vi "LV connector pane.vi"(8 "error in (no error)":errorcluster, 11 "reference":refnum<vi>) -> (0 "error out":errorcluster, 3 "conpane":string)   [LabVIEW 2012]
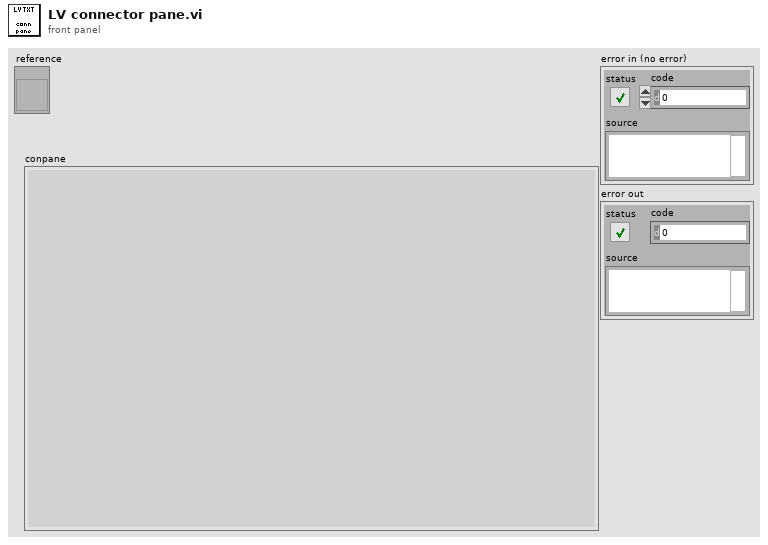
[diagram p1: front panel]
types:
  T1 = enum16{"Invalid Wire Rule", "Required", "Recommended", "Optional", "Dynamic Dispatch"}[]
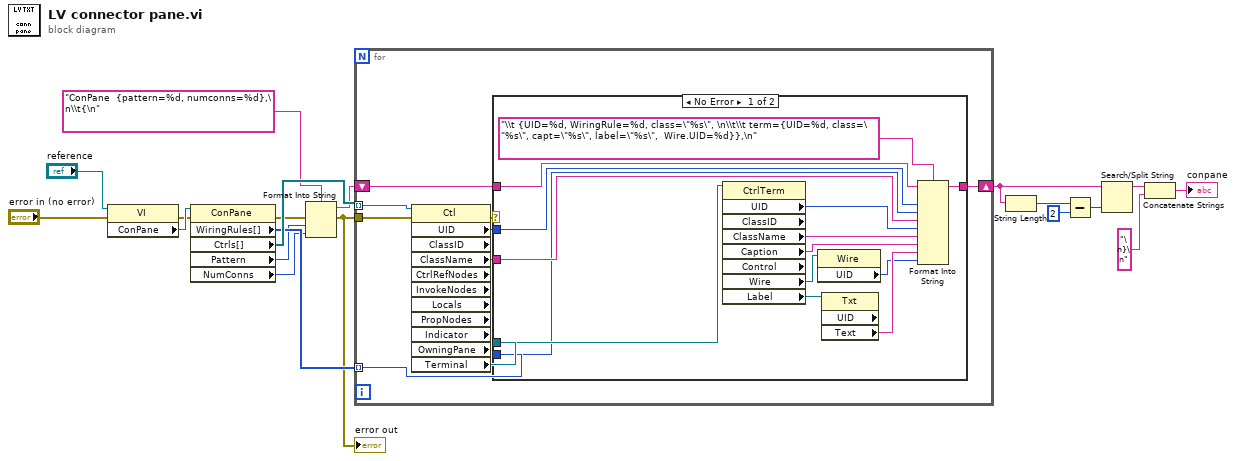
[diagram p0: block diagram]
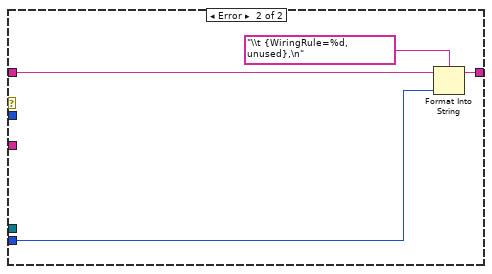
[diagram p2: hidden frame]
diagram:
  n1 = property class="VI"(reference="reference", error in="error in (no error)") -> (error out=w2:errorcluster, "ConPane"=w19:refnum<vi>)  [unwired: 1 out]
  n2 = property class="ConPane"(reference=w19, error in=w2) -> (error out=w5:errorcluster, "WiringRules[]"=w10:T1, "Ctrls[]"=w11:refnum<vi>[], "Pattern"=w8:u32, "NumConns"=w7:u32)  [unwired: 1 out]
  n3 = Format Into String(format string="ConPane  {pattern=%d, numconns=%d},\n\\t{\n", error in=w5, w8, w7) -> (resulting string=w6:string, error out=w1:errorcluster)  [unwired: 1 in]
  "error out" <- w1
  n4 = for {
    tunnel: w11 -> [w28] mode=indexing
    shift-right: [w23] -> w13
    shift-left: w6 -> [w26]
    tunnel: w10 -> [w21] mode=indexing
    tunnel: w1 -> [w27]
    n5 = property class="Ctl" props=["UID", "ClassID", "ClassName", "CtrlRefNodes", "InvokeNodes", "Locals", "PropNodes", "Indicator", "OwningPane", "Terminal"](reference=w28, error in=w27) -> (error out=w20:errorcluster, "UID"=w22:i32, "ClassName"=w25:string, "Terminal"=w24:refnum<vi>)  [unwired: 8 out]
    n6 = case shown="No Error" w20 {
      tunnel: w26 -> [w42 w44]
      tunnel: w25 -> [w40 _]
      tunnel: w24 -> [w39 _]
      tunnel: [w31 w43] -> w23
      tunnel: w22 -> [w30 _]
      tunnel: w21 -> [w29 w45]
      frame No Error {
        n7 = property class="CtrlTerm" props=["UID", "ClassID", "ClassName", "Caption", "Control", "Wire", "Label"](reference=w39) -> ("UID"=w36:i32, "ClassName"=w35:string, "Caption"=w34:string, "Wire"=w38:refnum<vi>, "Label"=w37:refnum<vi>)  [unwired: 1 in, 4 out]
        n8 = property class="Wire"(reference=w38) -> ("UID"=w32:i32)  [unwired: 1 in, 2 out]
        n9 = property class="Txt" props=["UID", "Text"](reference=w37) -> ("Text"=w33:string)  [unwired: 1 in, 3 out]
        n10 = Format Into String(format string="\\t {UID=%d, WiringRule=%d, class=\"%s\", \n\\t\\t term={UID=%d, class=\"%s\", capt=\"%s\", label=\"%s\",  Wire.UID=%d}},\n", initial string=w42, w30, w29, w40, w36, w35, w34, w33, w32) -> (resulting string=w31:string)  [unwired: 1 in, 1 out]
      }
      frame Error {
        n11 = Format Into String(format string="\\t {WiringRule=%d, unused},\n", initial string=w44, w45) -> (resulting string=w43:string)  [unwired: 1 in, 1 out]
      }
    }
  }
  n12 = String Length(string=w13) -> (length=w14:i32)
  n13 = Subtract(x=w14, y=2) -> (x-y=w16:i32)
  n14 = Search/Split String(string=w13, offset (0)=w16) -> (substring before match=w12:string)  [unwired: 1 in, 2 out]
  n15 = Concatenate Strings(w12, "\n}\n" ("format string")) -> (→"conpane":string)
